vi "Read Actor DVR.vi"(11 "TEMPLATE Actor in":refnum<class "{{Name}}Actor.lvclass">) -> ()   [LabVIEW 2020, in "_Template.lvlib" / "Templates.lvlib" / "{{Name}}Actor.lvlib" / "{{Name}}Actor.lvclass"]
uses:
  {{Name}}Actor.lvclass
  {{Name}}Actor.lvclass/{{Name}}Actor.ctl
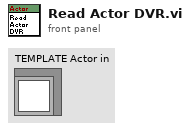
[diagram p1: front panel]
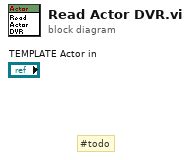
[diagram p0: block diagram]
diagram:
  # "#todo"
